vi "FIRE KICKER.vi"(8 "error in (no error)":errorcluster, 10 "delay seconds":dbl=1.67 format="%_5g", 11 "PhoenixMotorControlDevRef in":T1) -> (0 "error out":errorcluster, 3 "PhoenixMotorControlDevRef out":T1)   [LabVIEW 2020]
uses:
  <vilib>/Rock Robotics/WPI/MotorControl/WPI_MotorControlDeviceRef.ctl
  <vilib>/Rock Robotics/WPI/MotorControl/WPI_MotorControlType.ctl
  <vilib>/Rock Robotics/SystemInterfaces/DIO/FPGA_DIOPWMChannel.ctl
  <vilib>/Rock Robotics/WPI/PWM/WPI_PWMDeadband.ctl
  <vilib>/Rock Robotics/SystemInterfaces/DIO/FPGA_DIOChannel.ctl
  <vilib>/Rock Robotics/WPI/ThirdParty/Phoenix-LabVIEW/Motor Controller/Controls/CTRE_Phoenix_MotorControl_ControlMode.ctl
  <vilib>/Rock Robotics/Network Tables/NT Write Boolean.vi
  <vilib>/Rock Robotics/Network Tables/NT Read Boolean.vi
panel:
  # "Bosch seat motor runs at 24 rpm free at 100% = 0.4 rev/s\nthe 16/24 chain sprockets form a gear ratio of 0.667:1\ntherefore the wheel speed @ 100% will be 0.6 rev/s\n1 rev will take at least 1.67 s"
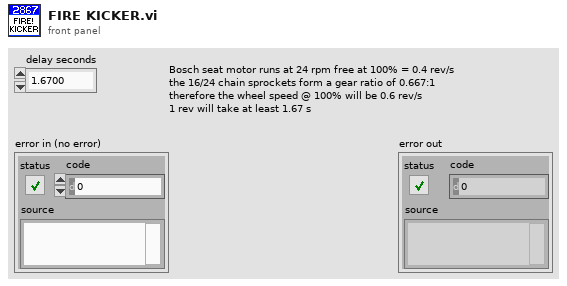
[diagram p1: front panel]
types:
  T1 = typedef "WPI_MotorControlDeviceRef.ctl" = cluster{"DeviceStatus":errorcluster, "Type":T2, "PWM":cluster{"PWM Channel":T3, "DeadBand":T4}, "CAN":cluster{"Device Number":u8, "SetOutput VI Ref":variant, "GetOutput VI Ref":variant, "Enable VI Ref":variant, "Disable VI Ref":variant, "Data":variant}, "Invert":bool, "DIO PWM":cluster{"PWM \"Enable\" Channel":T3, "DIOChannel":T5, "PWM Rate":dbl}}
  T2 = typedef "WPI_MotorControlType.ctl" = enum16{"PWM", "CAN", "DIO PWM"}
  T3 = typedef "FPGA_DIOPWMChannel.ctl" = enum8{"PWM 0", "PWM 1", "PWM 2", "PWM 3", "PWM 4", "PWM 5", "PWM 6", "PWM 7", "PWM 8", "PWM 9", "PWM MXP 0", "PWM MXP 1", "PWM MXP 2", "PWM MXP 3", "PWM MXP 4", "PWM MXP 5", "PWM MXP 6", "PWM MXP 7", "PWM MXP 8", "PWM MXP 9", "Invalid"}
  T4 = typedef "WPI_PWMDeadband.ctl" = cluster{"Name":string, "maxPositivePwm":i32, "minPositivePwm":i32, "centerPwm":i32, "maxNegativePwm":i32, "minNegativePwm":i32, "angularRange":u16}
  T5 = typedef "FPGA_DIOChannel.ctl" = enum8{"DIO 0", "DIO 1", "DIO 2", "DIO 3", "DIO 4", "DIO 5", "DIO 6", "DIO 7", "DIO 8", "DIO 9", "DIO MXP 0", "DIO MXP 1", "DIO MXP 2", "DIO MXP 3", "DIO MXP 4", "DIO MXP 5", "DIO MXP 6", "DIO MXP 7", "DIO MXP 8", "DIO MXP 9", "DIO MXP 10", "DIO MXP 11", "DIO MXP 12", "DIO MXP 13", "DIO MXP 14", "DIO MXP 15", "SPI Port CS1", "SPI Port CS2", "SPI Port CS3", "SPI Port MISO", "SPI Port MOSI", "Invalid"}
  T6 = typedef "CTRE_Phoenix_MotorControl_ControlMode.ctl" = u16
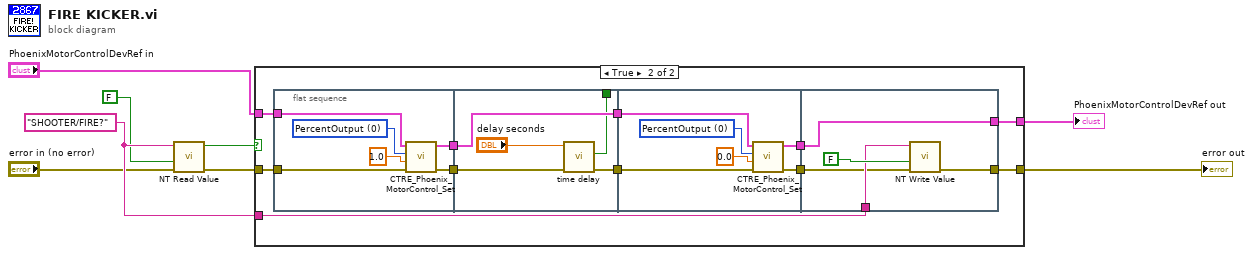
[diagram p0: block diagram]
diagram:
  w4 = "SHOOTER/FIRE?" ("string")
  n1 = call-poly <vilib>:"NT Read Value.vi"("error in"="error in (no error)", "Default Value"=FALSE, "Name"=w4) -> ("error out"=w2:errorcluster, "Boolean"=w5:bool)  [unwired: 7 in]
  n2 = case shown="True" w5 {
    tunnel: [w10 w15] -> w8
    tunnel: [w9 w14] -> w7
    tunnel: "PhoenixMotorControlDevRef in" -> [w10 w13]
    tunnel: w2 -> [w9 w12]
    tunnel: w4 -> [_ w11]
    frame False {
    }
    frame True {
      n3 = flat-sequence {
        tunnel: [w23] -> w21
        tunnel: [w22] -> w20
        tunnel: w12 -> [w26]
        tunnel: w13 -> [w24]
        tunnel: w21 -> [w30]
        tunnel: w20 -> [w32]
        tunnel: [w31] -> w19
        tunnel: [w30] -> w18
        tunnel: [w28] -> _
        tunnel: w19 -> [w36]
        tunnel: [w35] -> w17
        tunnel: w18 -> [w34]
        tunnel: [w33] -> w16
        tunnel: [w39] -> w14
        tunnel: w17 -> [w40]
        tunnel: [w43] -> w15
        tunnel: w16 -> [w43]
        tunnel: w11 -> [w41]
        frame #0 {
          w25 = T6 0 items=["PercentOutput"=0, "Position"=1, "Velocity"=2, "Current"=3, "Follower"=5, "MotionProfile"=6, "MotionMagic"=7, "MotionProfileArc"=10, "Disabled"=15] ("Control Mode")
          n4 = call <vilib>:"CTRE_Phoenix_MotorControl_Set.vi"("error in (no error)"=w26, "Output"=1.0, "Control Mode"=w25, "PhoenixMotorControlDevRef"=w24) -> ("error out"=w22:errorcluster, "PhoenixMotorControlDevRef"=w23:T1)  [unwired: 6 in]
        }
        frame #1 {
          n5 = call "time delay.vi"("error in (no error)"=w32, "timer delay (s)"="delay seconds") -> ("error out"=w31:errorcluster, "done?"=w28:bool)  [unwired: 8 in]
        }
        frame #2 {
          w37 = T6 0 items=["PercentOutput"=0, "Position"=1, "Velocity"=2, "Current"=3, "Follower"=5, "MotionProfile"=6, "MotionMagic"=7, "MotionProfileArc"=10, "Disabled"=15] ("Control Mode")
          n6 = call <vilib>:"CTRE_Phoenix_MotorControl_Set.vi"("error in (no error)"=w36, "Output"=0.0, "Control Mode"=w37, "PhoenixMotorControlDevRef"=w34) -> ("error out"=w35:errorcluster, "PhoenixMotorControlDevRef"=w33:T1)  [unwired: 6 in]
        }
        frame #3 {
          n7 = call-poly <vilib>:"NT Write Value.vi"("error in"=w40, "Boolean"=FALSE, "Name"=w41) -> ("error out"=w39:errorcluster)  [unwired: 8 in]
        }
      }
    }
  }
  "error out" <- w7
  "PhoenixMotorControlDevRef out" <- w8
